vi "Autonomous Setup Global Variable.vi"() -> ()   [LabVIEW 2015]
panel:
  in  "Taking Shot?":bool
  in  "Choose Goal":cluster{"High Goal":bool, "Low Goal":bool}
  in  "Choose Starting Position":T1
  in  "Choose Obstacle Type":T2
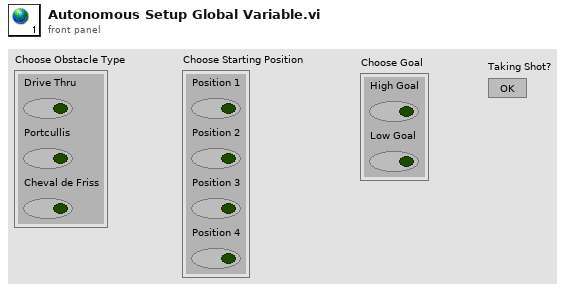
[diagram p1: front panel]
types:
  T1 = cluster{"Position 4":bool, "Position 3":bool, "Position 2":bool, "Position 1":bool}
  T2 = cluster{"Drive Thru":bool, "Portcullis":bool, "Cheval de Friss":bool}
diagram:
